vi "sv_Adjust Numeric String Precision.vi"(8 "error in (no error)":errorcluster, 9 "change in digits/precision":i32=-1, 10 "original format string":string="%.4f", 11 "numeric text":string="3.1416") -> (0 "error out":errorcluster, 2 "new format string":string)   [LabVIEW 2017]
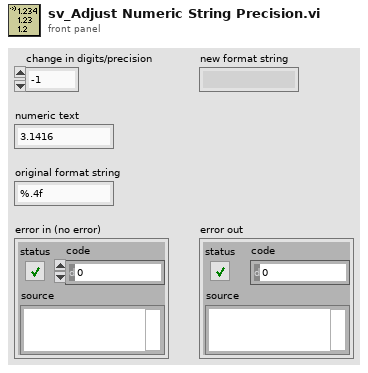
[diagram p1: front panel]
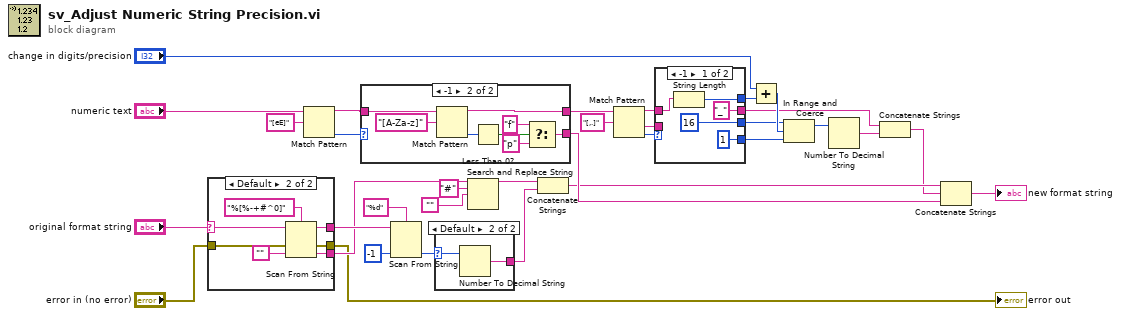
[diagram p0: block diagram]
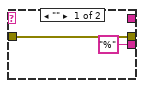
[diagram p2: hidden frame]
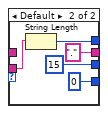
[diagram p3: hidden frame]
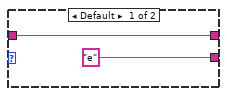
[diagram p4: hidden frame]
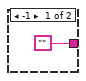
[diagram p5: hidden frame]
diagram:
  n1 = case shown="Default" "original format string" {
    selector: "original format string" -> [_ w38]
    tunnel: ["%" ("default value 1") w40] -> w10
    tunnel: [_ w39] -> w32
    tunnel: "error in (no error)" -> [w34 w37]
    tunnel: [w34 w36] -> w1
    frame "" {
    }
    frame Default {
      n2 = Scan From String(format string="%[%-+#^0]", input string=w38, error in=w37, default 1="" ("default value 1")) -> (remaining string=w39:string, error out=w36:errorcluster, output 1=w40:string)  [unwired: 1 in, 1 out]
    }
  }
  "error out" <- w1
  n3 = Match Pattern(string="numeric text", regular expression="[eE]") -> (before substring=w14:string, offset past match=w13:i32)  [unwired: 1 in, 2 out]
  n4 = case shown="-1" w13 {
    tunnel: ["e" ("t") w45] -> w29
    tunnel: w14 -> [w43 w51]
    tunnel: [w43 w50] -> w19
    frame Default {
    }
    frame -1 {
      n5 = Match Pattern(string=w51, regular expression="[A-Za-z]") -> (before substring=w50:string, offset past match=w49:i32)  [unwired: 1 in, 2 out]
      n6 = Less Than 0?(x=w49) -> (x < 0?=w47:bool)
      n7 = Select(t="f" ("regular expression"), s=w47, f="p") -> (s? t:f=w45:string)
    }
  }
  n8 = Scan From String(format string="%d", input string=w32, default 1=-1 ("default value 1")) -> (output 1=w5:i32)  [unwired: 2 in, 3 out]
  n9 = case shown="Default" w5 {
    selector: w5 -> [_ w54]
    tunnel: ["" w55] -> w28
    frame -1 {
    }
    frame Default {
      n10 = Number To Decimal String(number=w54) -> (decimal integer string=w55:string)  [unwired: 1 in]
    }
  }
  n11 = Search and Replace String(input string=w10, search string="#", replace string="" ("replace string (\"\")")) -> (result string=w11:string)  [unwired: 5 in, 3 out]
  n12 = Concatenate Strings(w11, w28) -> (w8:string)
  n13 = Match Pattern(string=w19, regular expression="[,.]") -> (before substring=w18:string, after substring=w15:string, offset past match=w17:i32)  [unwired: 1 in, 1 out]
  n14 = case shown="-1" w17 {
    tunnel: w15 -> [_ w65]
    tunnel: [w59 w63] -> w20
    tunnel: w18 -> [w60 _]
    tunnel: ["_" ("format string") "." ("search string")] -> w22
    tunnel: [16 ("default value 1") 15 ("default value 1")] -> w23
    tunnel: [1 ("default value 1") 0 ("default value 1")] -> w24
    frame -1 {
      n15 = String Length(string=w60) -> (length=w59:i32)
    }
    frame Default {
      n16 = String Length(string=w65) -> (length=w63:i32)
    }
  }
  n17 = Add(x="change in digits/precision", y=w20) -> (x+y=w26:i32)
  n18 = In Range and Coerce(upper limit=w23, x=w26, lower limit=w24) -> (coerced(x)=w25:i32)  [unwired: 1 out]
  n19 = Number To Decimal String(number=w25) -> (decimal integer string=w6:string)  [unwired: 1 in]
  n20 = Concatenate Strings(w22, w6) -> (w7:string)
  n21 = Concatenate Strings(w8, w7, w29) -> (→"new format string":string)
